vi "Logging Get Remote Log.vi"(4 "error in (no error)":errorcluster, 5 "Host":string, 6 "Name":string, 7 "Path":path=path "c:/logs") -> (0 "error out":errorcluster, 2 "Name Out":string, 3 "Path out":path)   [LabVIEW 2012, in "femtoRoboLib.lvlib"]
uses:
  femtoRoboLib.lvlib
  <vilib>/FTP/NI_FTP.lvlib
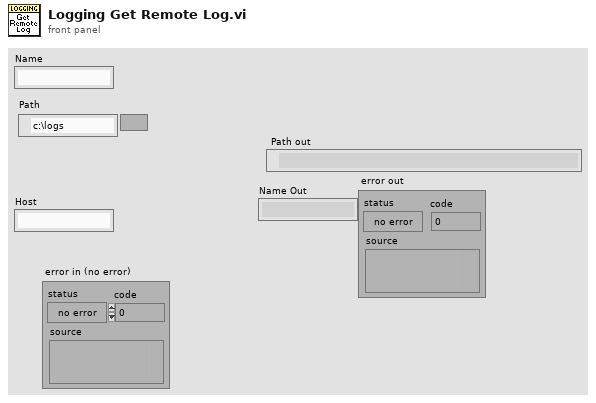
[diagram p1: front panel]
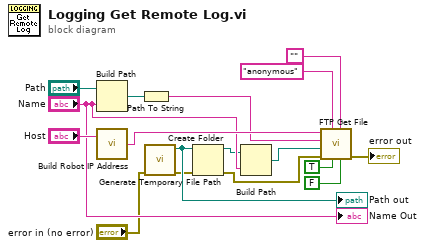
[diagram p0: block diagram]
diagram:
  n1 = Build Path(base path="Path", name or relative path="Name") -> (appended path=w13:path)
  n2 = call "Build Robot IP Address.vi"("In Address"="Host") -> ("Out Address"=w16:string)  [unwired: 1 in]
  n3 = Path To String(path=w13) -> (string=w12:string)
  n4 = call <vilib>:"Generate Temporary File Path.vi"("error in (no error)"="error in (no error)") -> ("error out"=w3:errorcluster, "Unique Temporary File Path"=w6:path)  [unwired: 9 in]
  "Path out" <- w6
  n5 = Create Folder(path (use dialog)=w6, error in=w3) -> (created path=w5:path, error out=w2:errorcluster)  [unwired: 1 in, 1 out]
  n6 = Build Path(base path=w5, name or relative path="Name") -> (appended path=w8:path)
  n7 = call <vilib>:"FTP Get File.vi"("active (T)"=FALSE, "password"="", "binary (F)"=TRUE, "user"="anonymous", "error in (no error)"=w2, "local path"=w8, "remote path"=w12, "host"=w16) -> ("error out"=→"error out":errorcluster)  [unwired: 2 in, 1 out]
  "Name Out" <- "Name"
